vi "Event-Display-refresh.vi"(7 "Display refresh":bool, 8 "error in (no error)":errorcluster, 10 "Data ref. in":refnum<data-value>, 11 "UI ref. in":refnum<data-value>) -> (0 "error out":errorcluster, 2 "Data ref.":refnum<data-value>, 3 "UI ref.":refnum<data-value>)   [LabVIEW 2013, in "CameraVision.lvlib" / "CV-UI.lvclass"]
uses:
  CV-UI.lvclass
  Main/CV-Main.lvclass
  Main/Main-actions.ctl
  Control-names.ctl
  CV-UI.lvclass/CV-UI.ctl
  Read Image refresh.vi
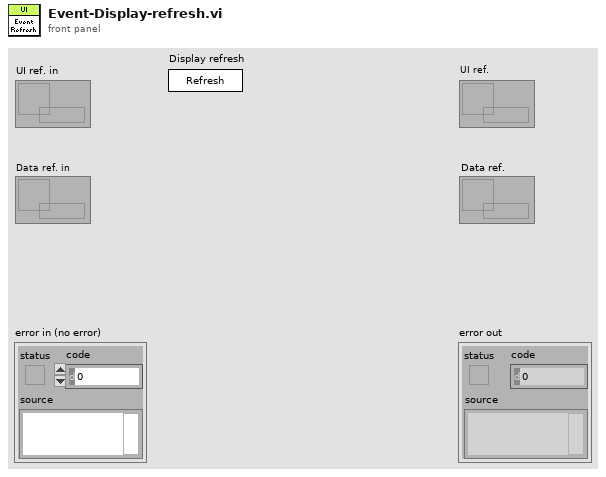
[diagram p1: front panel]
types:
  T1 = typedef "CameraVision.lvlib/CV-UI.lvclass/Control-names.ctl" = enum16{"Start acquisition", "Activate", "Stop acquisition", "Settings type", "Load settings", "Save settings", "Import images", "Camera selector", "Image type selector", "Batch browser", "Image refresh", "Parameter tabs", "Displays", "Processing tabs", "Processing selector", "Map characteristic", "Show info", "Manual trigger"}
  T2 = typedef "CameraVision.lvlib/CV-Main.lvclass/Main-actions.ctl" = enum16{"Idle", "Initialize", "Load defaults", "Update settings", "Check settings", "Save settings", "Save settings with dialog", "Load settings", "Load data", "Activate", "Start", "Wait for start signal", "Acquire & process", "Iterate", "Stop", "Refresh display", "Refresh status", "View camera settings", "View grabber settings", "Exit"}
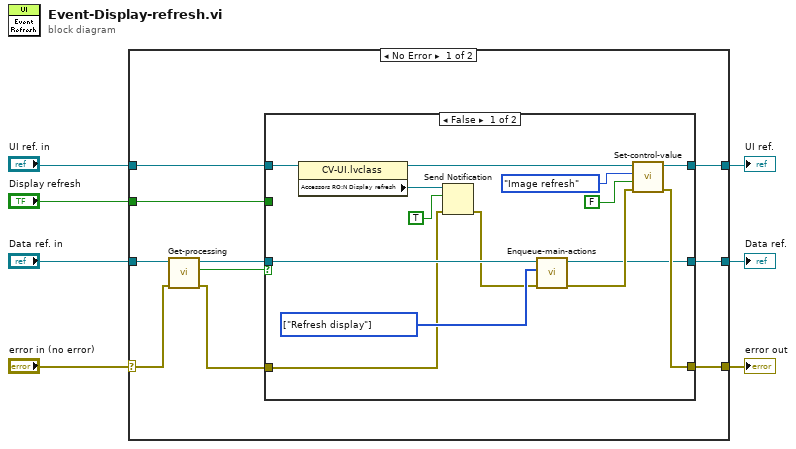
[diagram p0: block diagram]
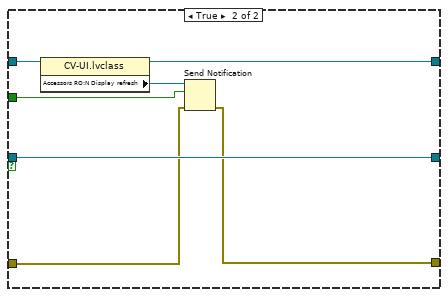
[diagram p2: hidden frame]
diagram:
  n1 = case shown="No Error" "error in (no error)" {
    selector: "error in (no error)" -> [w11 w41]
    tunnel: [w12 w41] -> w6
    tunnel: [w14 w40] -> w4
    tunnel: "UI ref. in" -> [w10 w40]
    tunnel: "Data ref. in" -> [w17 w39]
    tunnel: "Display refresh" -> [w9 _]
    tunnel: [w13 w39] -> w1
    frame No Error {
      n2 = call "Get-processing.vi"("error in (no error)"=w11, "Data ref. in"=w17) -> ("error out"=w8:errorcluster, "Processing?"=w15:bool, "Data ref."=w16:refnum<data-value>)  [unwired: 7 in]
      n3 = case shown="False" w15 {
        tunnel: w10 -> [w22 w36]
        tunnel: w16 -> [w26 w38]
        tunnel: [w30 w35] -> w14
        tunnel: [w25 w38] -> w13
        tunnel: w8 -> [w19 w32]
        tunnel: [w28 w33] -> w12
        tunnel: w9 -> [_ w34]
        frame False {
          w31 = T2[] [enum."Refresh display"] items=["Idle", "Initialize", "Load defaults", "Update settings", "Check settings", "Save settings", "Save settings with dialog", "Load settings", "Load data", "Activate", "Start", "Wait for start signal", "Acquire & process", "Iterate", "Stop", "Refresh display", "Refresh status", "View camera settings", "View grabber settings", "Exit"] ("State array")
          n4 = property class="CV-UI.lvclass"(reference=w22) -> (reference out=w21:refnum<data-value>, "Accessors RO:N Display refresh"=w23:refnum<notifier>)  [unwired: 1 in, 1 out]
          n5 = Send Notification(notification=TRUE, notifier=w23, error in (no error)=w19) -> (error out=w20:errorcluster)  [unwired: 1 out]
          n6 = call "Enqueue-main-actions.vi"("error in (no error)"=w20, "State array"=w31, "Data ref. in"=w26) -> ("error out"=w29:errorcluster, "Data ref."=w25:refnum<data-value>)  [unwired: 6 in, 1 out]
          n7 = call "Set-control-value.vi"("error in (no error)"=w29, "Value"=FALSE ("Display refresh"), "Control name"=Control-names."Image refresh", "UI ref. in"=w21) -> ("error out"=w28:errorcluster, "UI ref."=w30:refnum<data-value>)  [unwired: 6 in]
        }
        frame True {
          n8 = property class="CV-UI.lvclass"(reference=w36) -> (reference out=w35:refnum<data-value>, "Accessors RO:N Display refresh"=w37:refnum<notifier>)  [unwired: 1 in, 1 out]
          n9 = Send Notification(notification=w34, notifier=w37, error in (no error)=w32) -> (error out=w33:errorcluster)  [unwired: 1 out]
        }
      }
    }
    frame Error {
    }
  }
  "error out" <- w6
  "Data ref." <- w1
  "UI ref." <- w4
